vi "Job (Caraya Test).vi"() -> ()   [LabVIEW 2013]
uses:
  <vilib>/LabVIEW Open Source Project/Cron Scheduler/Job/Job.lvclass
  Caraya Job Configuration -- cluster.ctl
  <vilib>/LabVIEW Open Source Project/Cron Scheduler/Job/Job.lvclass/Job.ctl
  <vilib>/LabVIEW Open Source Project/Cron Scheduler/Job/Read Abort Notifier.vi
  <vilib>/addons/_JKI Toolkits/Caraya/run-tests/Run Test (Scalar Path).vi
  <vilib>/addons/_JKI Toolkits/Caraya/Caraya.lvlib
  <vilib>/addons/_JKI.lib/Serialization/JSON/JKI JSON Serialization.lvlib
panel:
  out "Test Configuration":T1={"Test Path"=path "", "Report Path"=path "", "Inspect Recursively"=TRUE, "Verbose"=TRUE}
  out "Job out":refnum<class "Job.lvclass">
  out "error out":errorcluster
  in  "Job":refnum<class "Job.lvclass">
  out "stdout":string
  in  "stdin":string
  # "Macro: Initialize\nList the tasks to be execute for this job\n\nThere are two ways to terminate the job: \n1- Call the \"Macro: Exit\" state at the end of your task execution.\n2- Comment out the \"Macro: Exit\" state in \"Macro: Initialize\" case and monitor a Job completion condition instead. Use the \"Action: Check Job Complete\" state to instruct the job to terminate.\n\nAction: Read Standard Input\nUse this case to read the stdin terminal and initialize your job.\n\nAction: Write Standard Output\nMake sure to write your return value to the stdout terminal before exiting this VI."
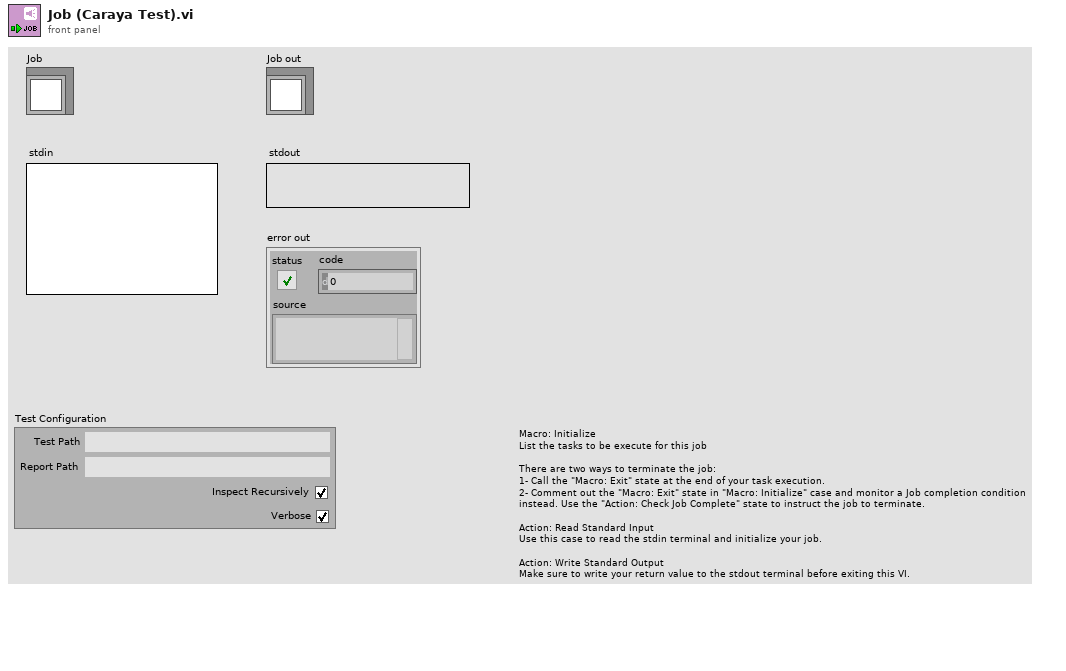
[diagram p1: front panel]
types:
  T1 = typedef "Caraya Job Configuration -- cluster.ctl" = cluster{"Test Path":path, "Report Path":path, "Inspect Recursively":bool, "Verbose":bool}
  T2 = enum32{"Invalid", "Standard", "Closed", "Hidden", "Minimized", "Maximized"}
  T3 = enum32{"invalid app kind", "Development System", "Run Time System", "Student Edition", "Embedded LabVIEW", "Evaluation", "Custom"}
  T4 = cluster{"Core":cluster{"Current VI Reference":refnum<vi>, "Close Panel on Exit?":bool}, "Job":refnum<class "Job.lvclass">, "stdin":string, "stdout":string, "stderror":errorcluster, "start time":timestamp, "Test Configuration":T1}
  T5 = cluster{"Current VI Reference":refnum<vi>, "Close Panel on Exit?":bool}
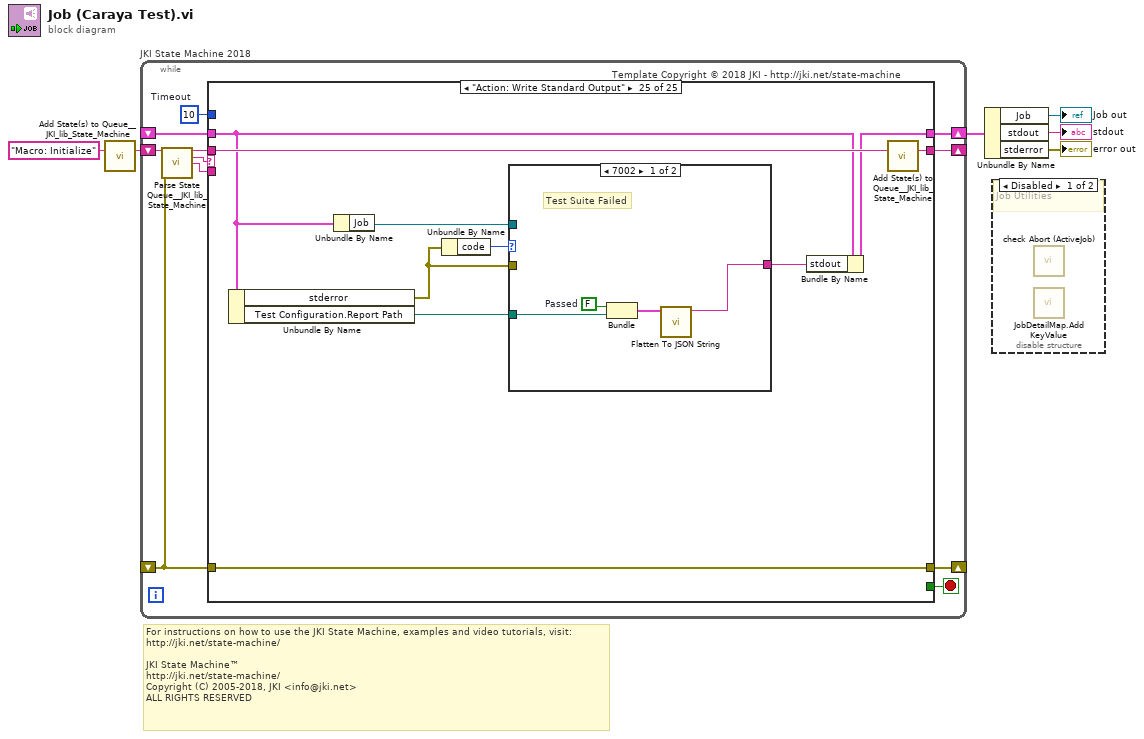
[diagram p0: block diagram]
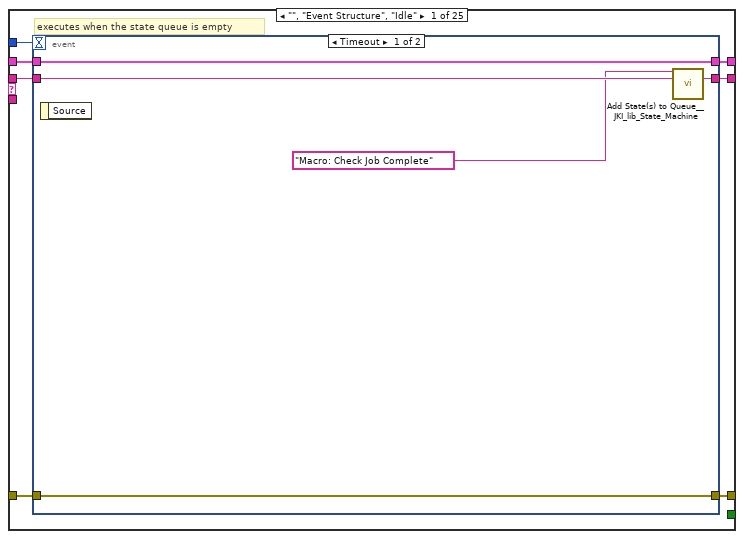
[diagram p3: hidden frame]
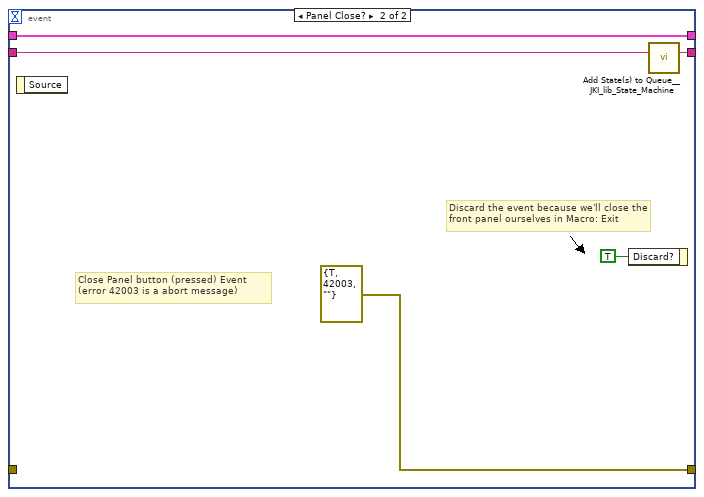
[diagram p4: hidden frame]
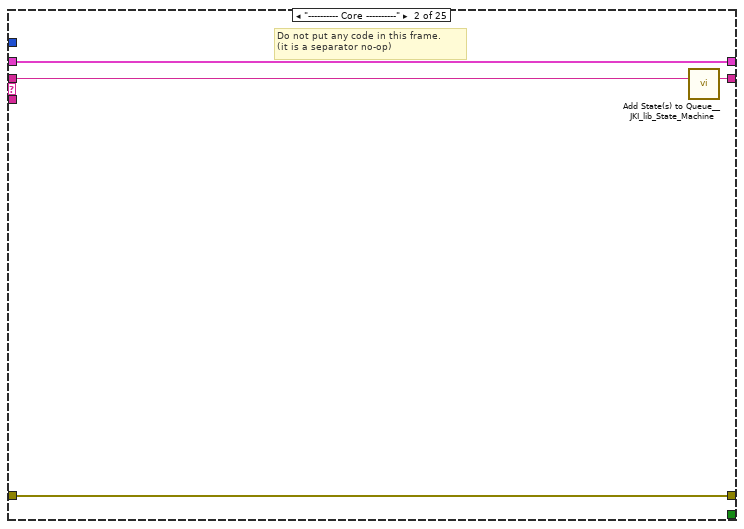
[diagram p5: hidden frame]
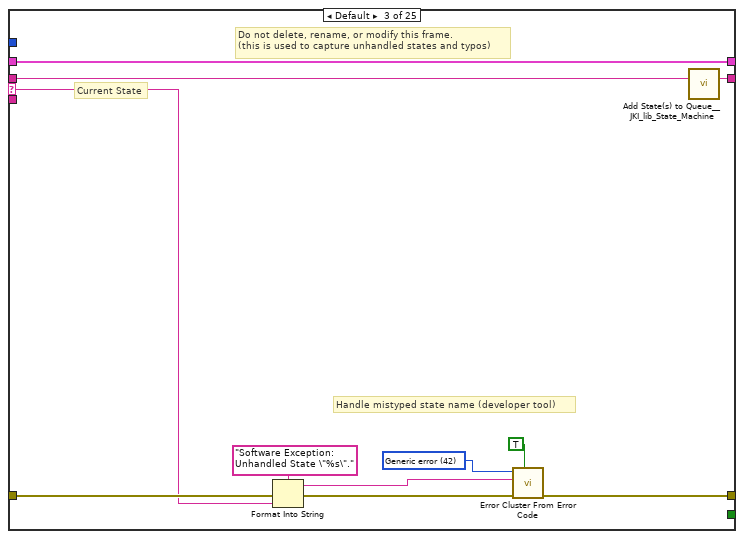
[diagram p6: hidden frame]
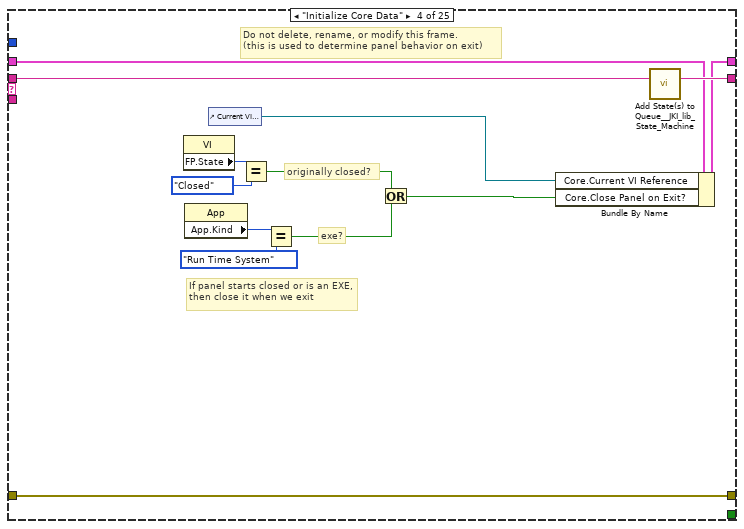
[diagram p7: hidden frame]
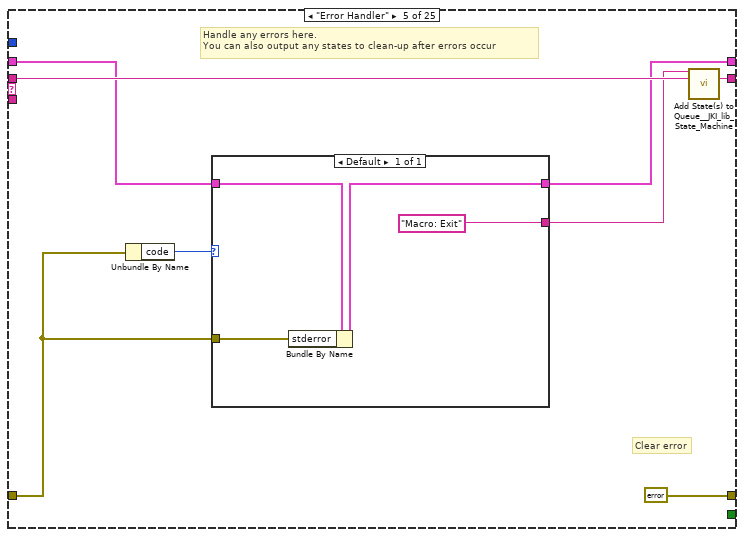
[diagram p8: hidden frame]
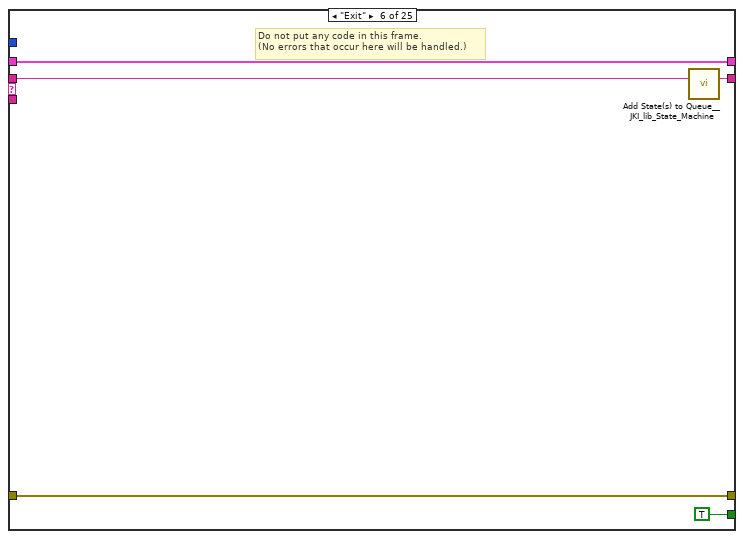
[diagram p9: hidden frame]
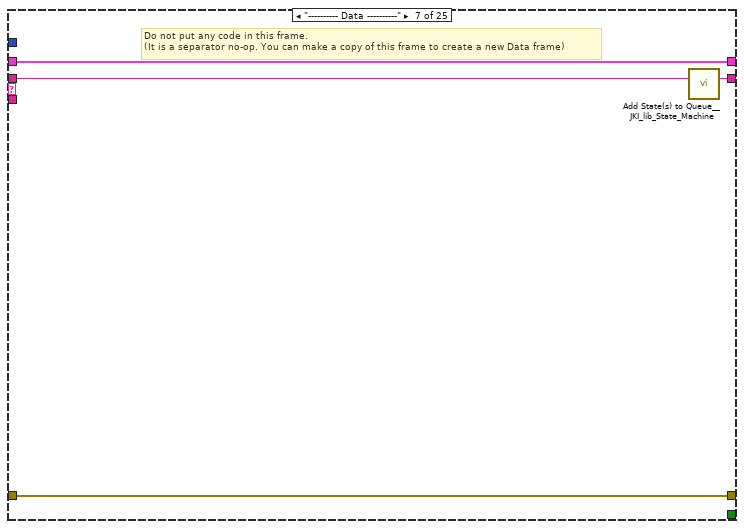
[diagram p10: hidden frame]
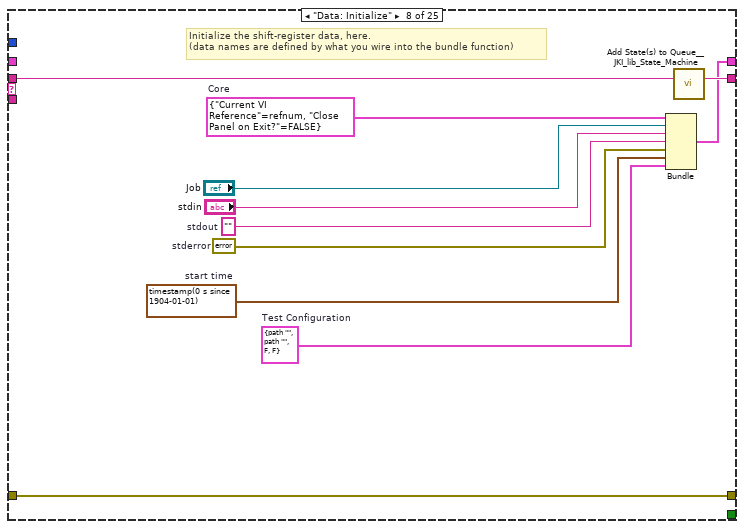
[diagram p11: hidden frame]
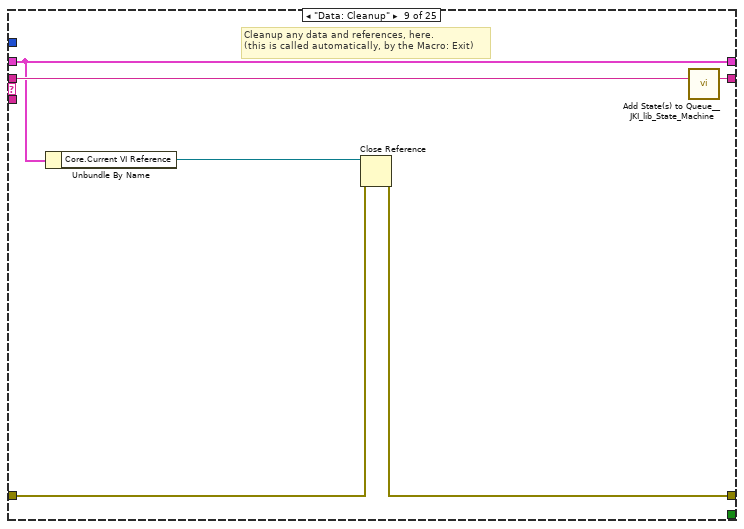
[diagram p12: hidden frame]
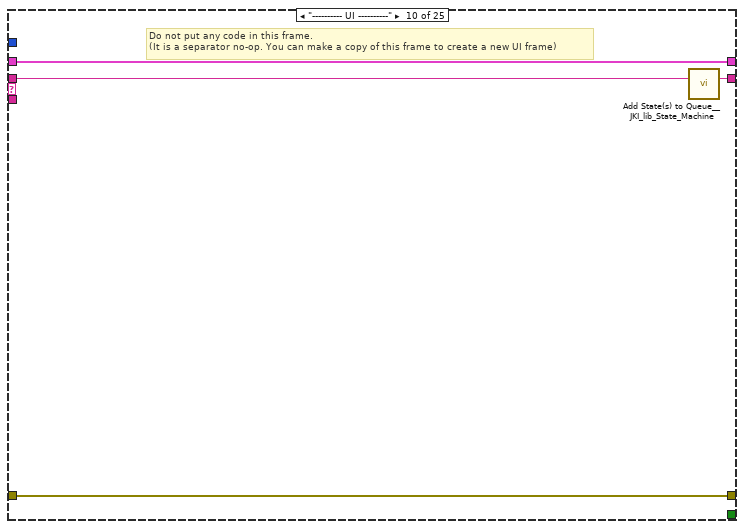
[diagram p13: hidden frame]
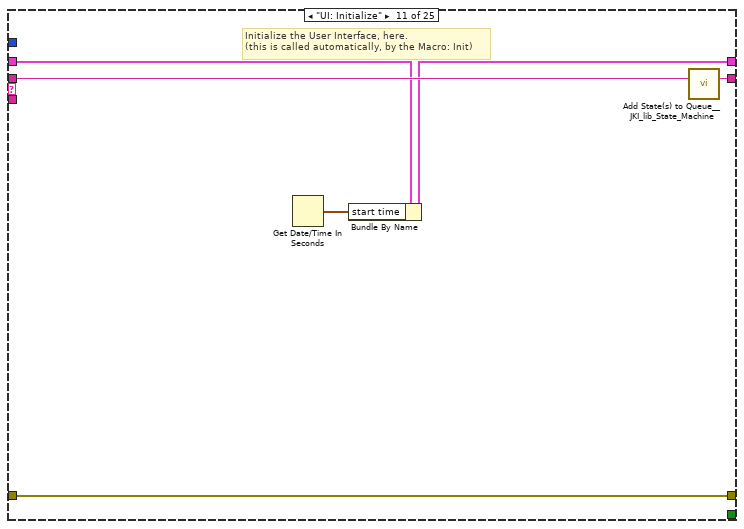
[diagram p14: hidden frame]
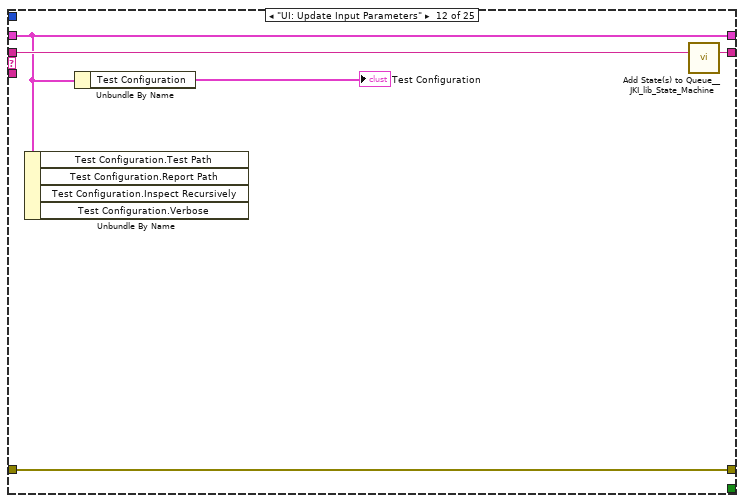
[diagram p15: hidden frame]
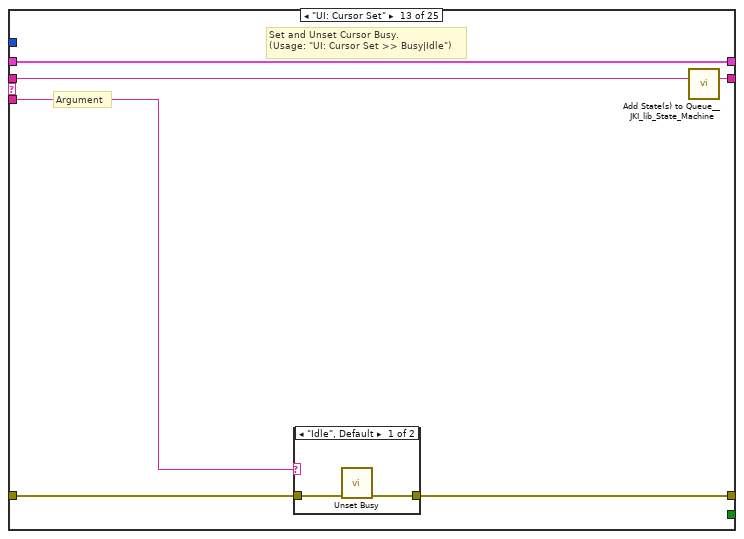
[diagram p16: hidden frame]
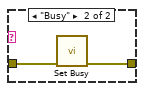
[diagram p17: hidden frame]
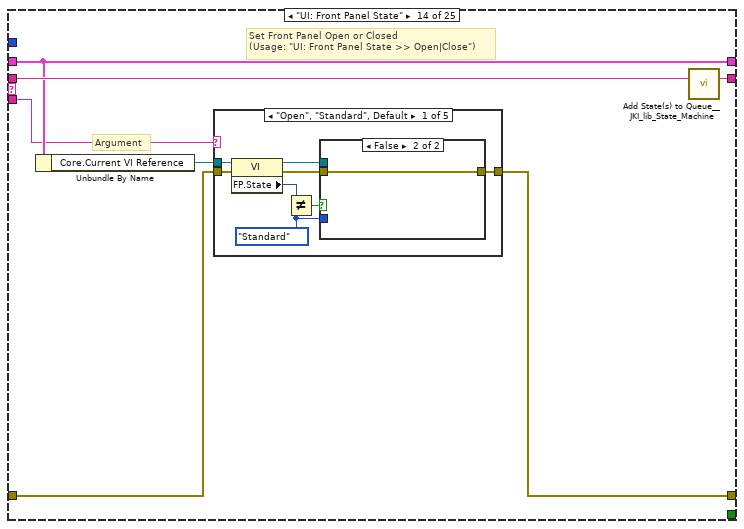
[diagram p18: hidden frame]
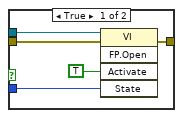
[diagram p19: hidden frame]
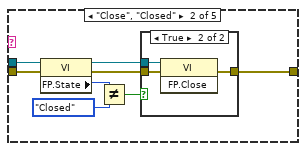
[diagram p20: hidden frame]
diagram:
  # "For instructions on how to use the JKI State Machine, examples and video tutorials, visit:\nhttp://jki.net/state-machine/\n\nJKI State Machine™\nhttp://jki.net/state-machine/\nCopyright (C) 2005-2018, JKI <info@jki.net>\nALL RIGHTS RESERVED"
  n1 = call <vilib>:"Add State(s) to Queue__JKI_lib_State_Machine.vi"("State(s) in (\"\")"="Macro: Initialize") -> ("States Out"=w6:string)  [unwired: 14 in]
  n2 = while "JKI State Machine 2018" {
    shift-right: [w10] -> w4
    shift-left: _ -> [w9]
    shift-right: [w13] -> _
    shift-left: _ -> [w7]
    shift-right: [w12] -> _
    shift-left: w6 -> [w14]
    stop <- w11 stop-if-true
    w8 = 10  # Timeout
    # "Template Copyright © 2018 JKI - http://jki.net/state-machine"
    n3 = call <vilib>:"Parse State Queue__JKI_lib_State_Machine.vi"("State Queue"=w14, "Error In (no error)"=w7) -> ("Remaining States"=w16:string, "Current State"=w17:string, "Arguments"=w15:string)  [unwired: 11 in]
    n4 = case shown="\"Action: Write Standard Output\"" w17 {
      selector: w17 -> [_ _ w39 _ _ _ _ _ _ _ _ _ _ _ _ _ _ _ _ w244 _ _ _ _ _]
      tunnel: w16 -> [w24 w38 w43 w62 w70 w79 w83 w94 w100 w104 w110 w115 w121 w132 w201 w206 w211 w222 w228 w248 w262 w272 w282 w307 w317]
      tunnel: w15 -> [_ _ _ _ _ _ _ _ _ _ _ _ w116 w126 _ _ _ _ _ _ _ _ _ _ _]
      tunnel: w9 -> [w22 w35 w41 w55 w65 w77 w80 _ w95 w101 w106 w112 w119 w128 w198 w203 w208 w219 w225 w242 w254 w270 w280 w305 w311]
      tunnel: [w21 w36 w45 w59 errorcluster {"status"=FALSE, "code"=0, "source"=""} ("error out") w76 w81 w91 w96 w102 w108 w113 w117 w129 w199 w204 w209 w220 w226 w229 w260 w264 w274 w288 w315] -> w13
      tunnel: w7 -> [w20 w36 w44 w59 w66 w76 w81 w91 w97 w102 w108 w113 w118 w130 w199 w204 w209 w220 w226 w233 w260 w263 w275 w283 w315]
      tunnel: [w23 w37 w42 w61 w69 w78 w82 w93 w99 w103 w109 w114 w120 w131 w200 w205 w210 w221 w227 w247 w261 w271 w281 w306 w316] -> w12
      tunnel: [_ _ _ _ _ TRUE _ _ _ _ _ _ _ _ _ _ _ _ _ _ _ _ _ _ _] -> w11
      tunnel: [w19 w35 w41 w60 w64 w77 w80 w92 w95 w101 w105 w112 w119 w128 w198 w203 w208 w219 w224 w246 w259 w269 w279 w304 w314] -> w10
      tunnel: w8 -> [w18 _ _ _ _ _ _ _ _ _ _ _ _ _ _ _ _ _ _ _ _ _ _ _ _]
      frame "", "Event Structure", "Idle" {
        # "executes when the state queue is empty"
        n5 = event shown="[0] Timeout" {
          selector: _ -> [_ _]
          dyn-events: _ -> [_ _]
          timeout: w18 -> [_ _]
          tunnel: w24 -> [w29 w34]
          tunnel: [w28 w33] -> w23
          tunnel: w22 -> [w26 w32]
          tunnel: [w27 errorcluster {"status"=TRUE, "code"=42003, "source"=""} ("error constant")] -> w21
          tunnel: w20 -> [w27 _]
          tunnel: [w26 w32] -> w19
          event Timeout {
            n6 = event-data() -> ()  [unwired: 1 in, 1 out]
            n7 = call <vilib>:"Add State(s) to Queue__JKI_lib_State_Machine.vi"("State(s) in Front (\"\")"="Macro: Check Job Complete", "State(s) in (\"\")"=w29) -> ("States Out"=w28:string)  [unwired: 13 in]
          }
          event Panel Close? {
            # "Discard the event because we'll close the front panel ourselves in Macro: Exit"
            # "Close Panel button (pressed) Event\n(error 42003 is a abort message)"
            n8 = event-data() -> ()  [unwired: 1 in, 1 out]
            n9 = event-data("Discard?"=TRUE) -> ()  [unwired: 1 in, 1 out]
            n10 = call <vilib>:"Add State(s) to Queue__JKI_lib_State_Machine.vi"("State(s) in (\"\")"=w34) -> ("States Out"=w33:string)  [unwired: 14 in]
          }
        }
      }
      frame "---------- Core ----------" {
        # "Do not put any code in this frame.\n(it is a separator no-op)"
        n11 = call <vilib>:"Add State(s) to Queue__JKI_lib_State_Machine.vi"("State(s) in (\"\")"=w38) -> ("States Out"=w37:string)  [unwired: 14 in]
      }
      frame Default {
        w48 = 42 items=["No error", "Argument error", "Memory is full", "Out of zone", "End of file", "File already open", "Generic file I/O error", "File not found", "File permission error", "Disk is full", "Duplicate path", "Too many files open", "System feature not enabled", "Resource file not found", "Cannot add resource", "Resource not found", "Image not found", "Image memory error", "Pen does not exist", "Config type invalid", "Config token not found", "Config parse error", "Config memory error", "Bad external code format", "Bad external code offset", "External code not present", "Null window", "Destroy window error", "Null menu", "Print aborted", "Bad print record", "Print driver error", "Windows error during printing", "Memory error during printing", "Print dialog error", "Generic print error", "Invalid device refnum", "Device not found", "Device parameter error", "Device unit error", "Cannot open device", "Device call aborted", "Generic error", "Cancelled by user", "Object ID too low", "Object ID too high", "Object not in heap", "Unknown heap", "Unknown object (invalid DefProc)", "Unknown object (DefProc not in table)", "Message out of range", "Invalid (null) method", "Unknown message", "Manager call not supported", "Bad address", "Network operation in progress", "Network operation timed out", "Connection is busy", "Network attribute not supported", "Network error", "Address in use", "System out of memory", "Connection aborted", "Connection refused", "Not connected", "Already connected", "Connection closed", "Initialization error (interapplication manager)", "Bad occurrence", "Wait on unbound occurrence handler", "Occurrence queue overflow", "Datalog type conflict", "Unused", "Unrecognized type (interapplication manager)", "Memory corrupt", "Failed to make temporary DLL", "Old CIN version", "Drag socket not found", "Failed to load drop-object", "Failed to register OLE object", "Failed to release OLE object", "Format specifier type mismatch", "Unknown format specifier", "Too few format specifiers", "Too many format specifiers", "Scan failed", "Newer CIN version", "Error converting to variant", "Runtime menu error", "Password tampered", "Variant attribute not found", "Incompatible variant data type", "Event data is not available", "Event Store is not present", "Occurrence is not found", "Event Queue is not created", "Event info is not available", "Refnum passed is NULL", "Error retrieving Class GUID", "Error retrieving CoClass GUID", "Error retrieving TypeLib GUID.", "Bad built application magic bytes.", "Specific driver is different from the specific driver associated with the Logical Name.", "There is no session opened to the class driver.", "Max Error", "MAX - Error with config objects", "MAX - Error loading configuration", "MAX - Group not supported"]
        # "Current State"
        # "Do not delete, rename, or modify this frame.\n(this is used to capture unhandled states and typos)"
        # "Handle mistyped state name (developer tool)"
        n12 = Format Into String(format string="Software Exception: Unhandled State \"%s\"." ("message"), error in=w44, w39) -> (resulting string=w47:string, error out=w46:errorcluster)  [unwired: 1 in]
        n13 = call <vilib>:"Error Cluster From Error Code.vi"("show call chain? (False)"=TRUE, "error in (no error)"=w46, "error message (\"\")"=w47, "error code (0)"=w48) -> ("error out"=w45:errorcluster)  [unwired: 5 in]
        n14 = call <vilib>:"Add State(s) to Queue__JKI_lib_State_Machine.vi"("State(s) in (\"\")"=w43) -> ("States Out"=w42:string)  [unwired: 14 in]
      }
      frame "Initialize Core Data" {
        # "Do not delete, rename, or modify this frame.\n(this is used to determine panel behavior on exit)"
        # "originally closed?"
        # "exe?"
        # "If panel starts closed or is an EXE, then close it when we exit"
        n15 = property class="VI"() -> ("FP.State"=w52:T2)  [unwired: 2 in, 2 out]
        n16 = property class="App"() -> ("App.Kind"=w58:T3)  [unwired: 2 in, 2 out]
        n17 = control-ref of="Current VI Reference"() -> (w53:refnum<vi>)
        n18 = Equal?(x=w52, y=T2."Closed" ("Front Panel Window:State")) -> (x = y?=w50:bool)
        n19 = Equal?(x=w58, y=T3."Run Time System" ("Application:Kind")) -> (x = y?=w56:bool)
        n20 = Or(x=w50, y=w56) -> (x .or. y?=w54:bool)
        n21 = Bundle By Name(cluster=w55, "Core.Current VI Reference"=w53, "Core.Close Panel on Exit?"=w54) -> (w60:T4)
        n22 = call <vilib>:"Add State(s) to Queue__JKI_lib_State_Machine.vi"("State(s) in (\"\")"=w62) -> ("States Out"=w61:string)  [unwired: 14 in]
      }
      frame "Error Handler" {
        # "Handle any errors here.\nYou can also output any states to clean-up after errors occur"
        # "Clear error"
        n23 = Unbundle By Name(w66) -> ("code"=w67:i32)
        n24 = case shown="Default" w67 {
          tunnel: w66 -> [w73]
          tunnel: w65 -> [w74]
          tunnel: [w72] -> w64
          tunnel: ["Macro: Exit"] -> w63
          frame Default {
            n25 = Bundle By Name(cluster=w74, "stderror"=w73) -> (w72:T4)
          }
        }
        n26 = call <vilib>:"Add State(s) to Queue__JKI_lib_State_Machine.vi"("State(s) in Front (\"\")"=w63, "State(s) in (\"\")"=w70) -> ("States Out"=w69:string)  [unwired: 13 in]
      }
      frame "Exit" {
        # "Do not put any code in this frame.\n(No errors that occur here will be handled.)"
        n27 = call <vilib>:"Add State(s) to Queue__JKI_lib_State_Machine.vi"("State(s) in (\"\")"=w79) -> ("States Out"=w78:string)  [unwired: 14 in]
      }
      frame "---------- Data ----------" {
        # "Do not put any code in this frame.\n(It is a separator no-op. You can make a copy of this frame to create a new Data frame)"
        n28 = call <vilib>:"Add State(s) to Queue__JKI_lib_State_Machine.vi"("State(s) in (\"\")"=w83) -> ("States Out"=w82:string)  [unwired: 14 in]
      }
      frame "Data: Initialize" {
        w84 = T1 {"Test Path"=path "", "Report Path"=path "", "Inspect Recursively"=FALSE, "Verbose"=FALSE}  # Test Configuration
        w85 = timestamp(0 s since 1904-01-01)  # start time
        w86 = errorcluster {"status"=FALSE, "code"=0, "source"=""}  # stderror
        w87 = ""  # stdout
        w90 = T5 {"Current VI Reference"=refnum, "Close Panel on Exit?"=FALSE}  # Core
        # "Initialize the shift-register data, here.\n(data names are defined by what you wire into the bundle function)"
        n29 = Bundle("Core"=w90, "Job"="Job", "stdin"="stdin", "stdout"=w87, "stderror"=w86, "start time"=w85, "Test Configuration"=w84) -> (w92:T4)  [unwired: 1 in]
        n30 = call <vilib>:"Add State(s) to Queue__JKI_lib_State_Machine.vi"("State(s) in (\"\")"=w94) -> ("States Out"=w93:string)  [unwired: 14 in]
      }
      frame "Data: Cleanup" {
        # "Cleanup any data and references, here.\n(this is called automatically, by the Macro: Exit)"
        n31 = Unbundle By Name(w95) -> ("Core.Current VI Reference"=w98:refnum<vi>)
        n32 = Close Reference(reference=w98, error in (no error)=w97) -> (error out=w96:errorcluster)
        n33 = call <vilib>:"Add State(s) to Queue__JKI_lib_State_Machine.vi"("State(s) in (\"\")"=w100) -> ("States Out"=w99:string)  [unwired: 14 in]
      }
      frame "---------- UI ----------" {
        # "Do not put any code in this frame.\n(It is a separator no-op. You can make a copy of this frame to create a new UI frame)"
        n34 = call <vilib>:"Add State(s) to Queue__JKI_lib_State_Machine.vi"("State(s) in (\"\")"=w104) -> ("States Out"=w103:string)  [unwired: 14 in]
      }
      frame "UI: Initialize" {
        # "Initialize the User Interface, here.\n(this is called automatically, by the Macro: Init)"
        n35 = Get Date/Time In Seconds() -> (seconds since 1Jan1904=w107:timestamp)
        n36 = Bundle By Name(cluster=w106, "start time"=w107) -> (w105:T4)
        n37 = call <vilib>:"Add State(s) to Queue__JKI_lib_State_Machine.vi"("State(s) in (\"\")"=w110) -> ("States Out"=w109:string)  [unwired: 14 in]
      }
      frame "UI: Update Input Parameters" {
        n38 = Unbundle By Name(w112) -> ()  [unwired: 4 out]
        n39 = Unbundle By Name(w112) -> ("Test Configuration"=→"Test Configuration":T1)
        n40 = call <vilib>:"Add State(s) to Queue__JKI_lib_State_Machine.vi"("State(s) in (\"\")"=w115) -> ("States Out"=w114:string)  [unwired: 14 in]
      }
      frame "UI: Cursor Set" {
        # "Argument"
        # "Set and Unset Cursor Busy.\n(Usage: \"UI: Cursor Set >> Busy|Idle\")"
        n41 = case shown="\"Idle\", Default" w116 {
          tunnel: w118 -> [w123 w125]
          tunnel: [w122 w124] -> w117
          frame "Idle", Default {
            n42 = call <vilib>:"Unset Busy.vi"("error in (no error)"=w123) -> ("error out"=w122:errorcluster)  [unwired: 10 in]
          }
          frame "Busy" {
            n43 = call <vilib>:"Set Busy.vi"("error in (no error)"=w125) -> ("error out"=w124:errorcluster)  [unwired: 9 in, 1 out]
          }
        }
        n44 = call <vilib>:"Add State(s) to Queue__JKI_lib_State_Machine.vi"("State(s) in (\"\")"=w121) -> ("States Out"=w120:string)  [unwired: 14 in]
      }
      frame "UI: Front Panel State" {
        # "Argument"
        # "Set Front Panel Open or Closed\n(Usage: \"UI: Front Panel State >> Open|Close\")"
        n45 = Unbundle By Name(w128) -> ("Core.Current VI Reference"=w127:refnum<vi>)
        n46 = case shown="\"Open\", \"Standard\", Default" w126 {
          tunnel: w130 -> [w138 w153 w164 w177 w190]
          tunnel: [w140 w154 w166 w179 w192] -> w129
          tunnel: w127 -> [w139 w151 w165 w178 w191]
          frame "Open", "Standard", Default {
            w133 = T2."Standard" ("State")
            n47 = property class="VI"(reference=w139, error in=w138) -> (reference out=w136:refnum<vi>, error out=w137:errorcluster, "FP.State"=w135:T2)
            n48 = Not Equal?(x=w135, y=w133) -> (x != y?=w134:bool)
            n49 = case shown="False" w134 {
              tunnel: [w144 w146] -> w140
              tunnel: w137 -> [w143 w146]
              tunnel: w136 -> [w142 _]
              tunnel: w133 -> [w141 _]
              frame True {
                n50 = invoke class="VI" method="FP.Open"(reference=w142, error in=w143, "Activate"=TRUE, "State"=w141) -> (error out=w144:errorcluster)  [unwired: 1 in, 4 out]
              }
              frame False {
              }
            }
          }
          frame "Close", "Closed" {
            n51 = property class="VI"(reference=w151, error in=w153) -> (reference out=w150:refnum<vi>, error out=w152:errorcluster, "FP.State"=w148:T2)
            n52 = Not Equal?(x=w148, y=T2."Closed" ("Front Panel Window:State")) -> (x != y?=w147:bool)
            n53 = case shown="True" w147 {
              tunnel: [w155 w158] -> w154
              tunnel: w152 -> [w155 w157]
              tunnel: w150 -> [_ w156]
              frame False {
              }
              frame True {
                n54 = invoke class="VI" method="FP.Close"(reference=w156, error in=w157) -> (error out=w158:errorcluster)  [unwired: 1 in, 2 out]
              }
            }
          }
          frame "Hidden", "Hide" {
            w159 = T2."Hidden" ("State")
            n55 = property class="VI"(reference=w165, error in=w164) -> (reference out=w162:refnum<vi>, error out=w163:errorcluster, "FP.State"=w161:T2)
            n56 = Not Equal?(x=w161, y=w159) -> (x != y?=w160:bool)
            n57 = case shown="True" w160 {
              tunnel: [w170 w171] -> w166
              tunnel: w163 -> [w169 w171]
              tunnel: w162 -> [w168 _]
              tunnel: w159 -> [w167 _]
              frame True {
                n58 = invoke class="VI" method="FP.Open"(reference=w168, error in=w169, "State"=w167) -> (error out=w170:errorcluster)  [unwired: 2 in, 4 out]
              }
              frame False {
              }
            }
          }
          frame "Minimize", "Minimized" {
            w172 = T2."Minimized" ("State")
            n59 = property class="VI"(reference=w178, error in=w177) -> (reference out=w175:refnum<vi>, error out=w176:errorcluster, "FP.State"=w174:T2)
            n60 = Not Equal?(x=w174, y=w172) -> (x != y?=w173:bool)
            n61 = case shown="True" w173 {
              tunnel: [w183 w184] -> w179
              tunnel: w176 -> [w182 w184]
              tunnel: w175 -> [w181 _]
              tunnel: w172 -> [w180 _]
              frame True {
                n62 = invoke class="VI" method="FP.Open"(reference=w181, error in=w182, "State"=w180) -> (error out=w183:errorcluster)  [unwired: 2 in, 4 out]
              }
              frame False {
              }
            }
          }
          frame "Maximize", "Maximized" {
            w185 = T2."Maximized" ("State")
            n63 = property class="VI"(reference=w191, error in=w190) -> (reference out=w188:refnum<vi>, error out=w189:errorcluster, "FP.State"=w187:T2)
            n64 = Not Equal?(x=w187, y=w185) -> (x != y?=w186:bool)
            n65 = case shown="True" w186 {
              tunnel: [w196 w197] -> w192
              tunnel: w189 -> [w195 w197]
              tunnel: w188 -> [w194 _]
              tunnel: w185 -> [w193 _]
              frame True {
                n66 = invoke class="VI" method="FP.Open"(reference=w194, error in=w195, "State"=w193) -> (error out=w196:errorcluster)  [unwired: 2 in, 4 out]
              }
              frame False {
              }
            }
          }
        }
        n67 = call <vilib>:"Add State(s) to Queue__JKI_lib_State_Machine.vi"("State(s) in (\"\")"=w132) -> ("States Out"=w131:string)  [unwired: 14 in]
      }
      frame "---------- Macro ----------" {
        # "Do not put any code in this frame.\n(It is a separator no-op. You can make a copy of this frame to create a new Macro frame)"
        n68 = call <vilib>:"Add State(s) to Queue__JKI_lib_State_Machine.vi"("State(s) in (\"\")"=w201) -> ("States Out"=w200:string)  [unwired: 14 in]
      }
      frame "Macro: Initialize" {
        w202 = "Data: Initialize\nInitialize Core Data\nUI: Initialize\nAction: Read Standard Input\nUI: Update Input Parameters\n\nUI: Front Panel State >> Open\n\n// Add your task actions below\nAction: Run Tests\n\nAction: Check Job Complete\n\n// Comment out the Macro: Exit line if you wish to exit on a condition\n// instead of exiting after a pre-determined action\n\n#Macro: Exit\n"  # Data: Initialize Initialize Core Data UI: Initialize Action: Read Standard Input UI: Update Input Parameters  UI: Front Panel State >> Open  // Add your task actions below Action: Run Tests  Action: Check Job Complete  // Comment out the Macro: Exit line if you wish to exit on a condition // instead of exiting after a pre-determined action  #Macro: Exit
        # "- Use the \"Action: Check Job Complete\" case to exit on a condition.\n- You can call Macro: Exit whenever you want to terminate the job.\n- Don't forget to set the Standard Output in the \"Action: Write Standard Output\" case if you wish to return results."
        # "Initialization Macro\n(This is called once, when the VI starts)"
        n69 = call <vilib>:"Add State(s) to Queue__JKI_lib_State_Machine.vi"("State(s) in Front (\"\")"=w202, "State(s) in (\"\")"=w206) -> ("States Out"=w205:string)  [unwired: 13 in]
      }
      frame "Macro: Check Job Complete" {
        # "Job Monitoring Macro\n(This is called regularly when the UI is idle)"
        n70 = call <vilib>:"Add State(s) to Queue__JKI_lib_State_Machine.vi"("State(s) in Front (\"\")"="Action: Check Job Complete\nAction: Check Abort", "State(s) in (\"\")"=w211) -> ("States Out"=w210:string)  [unwired: 13 in]
      }
      frame "Macro: Exit" {
        # "Exit Macro\n(This is called once, when the VI exits)"
        n71 = Unbundle By Name(w219) -> ("Core.Close Panel on Exit?"=w218:bool)
        n72 = Select(t="UI: Front Panel State >> Close", s=w218, f="") -> (s? t:f=w215:string)
        n73 = call <vilib>:"Add State(s) to Queue__JKI_lib_State_Machine.vi"("State(s) in Front (\"\")"="Action: Write Standard Output", "State(s) in (\"\")"=w215, "State(s) at Back (\"\")"="Data: Cleanup\nExit") -> ("States Out"=w213:string)  [unwired: 12 in]
        n74 = call <vilib>:"Add State(s) to Queue__JKI_lib_State_Machine.vi"("State(s) in Front (\"\")"=w213, "State(s) in (\"\")"=w222) -> ("States Out"=w221:string)  [unwired: 13 in]
      }
      frame "---------- Action ----------" {
        # "Action Separator\n(You can make a copy of, or modify, this frame)"
        n75 = Unbundle By Name(w225) -> ("Job"=w223:refnum<class "Job.lvclass">)  [unwired: 1 out]
        n76 = Bundle By Name(cluster=w225, "Job"=w223) -> (w224:T4)
        n77 = call <vilib>:"Add State(s) to Queue__JKI_lib_State_Machine.vi"("State(s) in (\"\")"=w228) -> ("States Out"=w227:string)  [unwired: 14 in]
      }
      frame "Action: Run Tests" {
        n78 = Unbundle By Name(w242) -> ("Job"=w245:refnum<class "Job.lvclass">)  [unwired: 1 out]
        n79 = Unbundle By Name(w242) -> ("Test Configuration.Report Path"=w237:path, "Test Configuration.Test Path"=w241:path, "Test Configuration.Inspect Recursively"=w239:bool, "Test Configuration.Verbose"=w238:bool)
        n80 = Get Date/Time In Seconds() -> (seconds since 1Jan1904=w243:timestamp)
        n81 = call <vilib>:"JobDetailMap.Add KeyValue.vi"("error in (no error)"=w233, "Value"=w243, "Key"=w244, "Job in"=w245) -> ("error out"=w232:errorcluster, "Job out"=w236:refnum<class "Job.lvclass">)  [unwired: 6 in]
        n82 = call-poly <vilib>:"Run Tests.vi"("Verbose"=w238, "Report Path"=w237, "Inspect Recursively (T)"=w239, "Test Path"=w241, "Interactive (T)"=FALSE) -> ("error out"=w230:errorcluster)  [unwired: 6 in]
        n83 = call <vilib>:"JobDetailMap.Add KeyValue.vi"("error in (no error)"=w232, "Value"=w230, "Key"="Post-Test Error", "Job in"=w236) -> ("error out"=w231:errorcluster, "Job out"=w235:refnum<class "Job.lvclass">)  [unwired: 6 in]
        n84 = Bundle By Name(cluster=w242, "Job"=w235) -> (w246:T4)
        n85 = Merge Errors(w231, w230) -> (w229:errorcluster)
        n86 = call <vilib>:"Add State(s) to Queue__JKI_lib_State_Machine.vi"("State(s) in (\"\")"=w248) -> ("States Out"=w247:string)  [unwired: 14 in]
      }
      frame "Action: Check Job Complete" {
        # "Terminates after a delay (demo).\nReplace with your own condition."
        n87 = Unbundle By Name(w254) -> ("Job"=w258:refnum<class "Job.lvclass">)
        n88 = Unbundle By Name(w254) -> ("start time"=w252:timestamp)
        n89 = Get Date/Time In Seconds() -> (seconds since 1Jan1904=w253:timestamp)
        n90 = Subtract(x=w253, y=w252) -> (x-y=w251:dbl)
        n91 = Bundle By Name(cluster=w254, "Job"=w258) -> (w259:T4)
        n92 = Greater Or Equal?(x=w251, y=3.0) -> (x >= y?=w249:bool)
        n93 = Select(t="Macro: Exit", s=w249, f="") -> (s? t:f=w255:string)
        n94 = call <vilib>:"Add State(s) to Queue__JKI_lib_State_Machine.vi"("State(s) in Front (\"\")"=w255, "State(s) in (\"\")"=w262) -> ("States Out"=w261:string)  [unwired: 13 in]
      }
      frame "Action: Check Abort" {
        n95 = Unbundle By Name(w270) -> ("Job"=w266:refnum<class "Job.lvclass">)  [unwired: 1 out]
        n96 = call <vilib>:"check Abort (ActiveJob).vi"("error in (no error)"=w263, "Job in"=w266) -> ("error out"=w267:errorcluster, "Abort"=w268:bool, "Job out"=w265:refnum<class "Job.lvclass">)  [unwired: 6 in, 1 out]
        n97 = Bundle By Name(cluster=w267, "status"=w268) -> (w264:errorcluster)
        n98 = Bundle By Name(cluster=w270, "Job"=w265) -> (w269:T4)
        n99 = call <vilib>:"Add State(s) to Queue__JKI_lib_State_Machine.vi"("State(s) in (\"\")"=w272) -> ("States Out"=w271:string)  [unwired: 14 in]
      }
      frame "Action: Update Map Data" {
        # "Use this pattern to add\nkey value pair data to the\nJob's map. This data is going\nto be available by the scheduler\nupon completion of the job."
        n100 = Unbundle By Name(w280) -> ("Job"=w278:refnum<class "Job.lvclass">)  [unwired: 1 out]
        n101 = Random Number (0-1)() -> (number: 0 to 1=w273:dbl)
        n102 = call <vilib>:"JobDetailMap.Add KeyValue.vi"("error in (no error)"=w275, "Value"=w273, "Key"="Value", "Job in"=w278) -> ("error out"=w274:errorcluster, "Job out"=w277:refnum<class "Job.lvclass">)  [unwired: 6 in]
        n103 = Bundle By Name(cluster=w280, "Job"=w277) -> (w279:T4)
        n104 = call <vilib>:"Add State(s) to Queue__JKI_lib_State_Machine.vi"("State(s) in (\"\")"=w282) -> ("States Out"=w281:string)  [unwired: 14 in]
      }
      frame "Action: Read Standard Input" {
        w292 = T1 {"Test Path"=path "", "Report Path"=path "", "Inspect Recursively"=FALSE, "Verbose"=FALSE}
        n105 = Unbundle By Name(w305) -> ("Job"=w303:refnum<class "Job.lvclass">, "stdin"=w296:string)
        n106 = call <vilib>:"Unflatten From JSON String.vi"("Nulls as Defaults (F)"=TRUE, "Type and Defaults"=w292, "error in (no error)"=w283, "JSON String"=w296) -> ("error out"=w294:errorcluster, "Variant"=w293:variant)  [unwired: 6 in]
        n107 = Variant To Data(error in=w294, type=w292, Variant=w293) -> (data=w291:T1, error out=w287:errorcluster)
        n108 = Unbundle By Name(w291) -> ("Test Path"=w300:path, "Report Path"=w299:path)
        n109 = Select(t="" ("Key"), s=w287, f="" ("Key")) -> (s? t:f=w284:string)
        n110 = call <vilib>:"JobDetailMap.Add KeyValue.vi"("Value"=w300, "Key"="Test Path", "Job in"=w303) -> ("error out"=w302:errorcluster, "Job out"=w301:refnum<class "Job.lvclass">)  [unwired: 7 in]
        n111 = call <vilib>:"JobDetailMap.Add KeyValue.vi"("error in (no error)"=w302, "Value"=w299, "Key"="Report Path", "Job in"=w301) -> ("error out"=w289:errorcluster, "Job out"=w297:refnum<class "Job.lvclass">)  [unwired: 6 in]
        n112 = Merge Errors(w283, w289) -> (w288:errorcluster)
        n113 = Bundle By Name(cluster=w305, "Job"=w297, "Test Configuration"=w291) -> (w304:T4)
        n114 = call <vilib>:"Add State(s) to Queue__JKI_lib_State_Machine.vi"("State(s) in Front (\"\")"=w284, "State(s) in (\"\")"=w307) -> ("States Out"=w306:string)  [unwired: 13 in]
      }
      frame "Action: Write Standard Output" {
        n115 = Unbundle By Name(w311) -> ("stderror"=w313:errorcluster, "Test Configuration.Report Path"=w308:path)
        n116 = Unbundle By Name(w311) -> ("Job"=w312:refnum<class "Job.lvclass">)
        n117 = Unbundle By Name(w313) -> ("code"=w309:i32)
        n118 = case shown="7002" w309 {
          selector: w309 -> [_ w329]
          tunnel: w313 -> [_ w332]
          tunnel: w312 -> [_ w331]
          tunnel: [w318 w330] -> w310
          tunnel: w308 -> [w319 w327]
          frame 7002 {
            w321 = FALSE  # Passed
            # "Test Suite Failed"
            n119 = Bundle("Passed"=w321, "Report Path"=w319) -> (w320:cluster{"Passed":bool, "Report Path":path})  [unwired: 1 in]
            n120 = call <vilib>:"Flatten To JSON String.vi"("Variant"=w320) -> ("JSON String"=w318:string)  [unwired: 9 in, 1 out]
          }
          frame Default {
            w328 = TRUE  # Passed
            n121 = call <vilib>:"Explain exception code.vi"("exception"=w329, "Job type"=w331) -> ("exception message"=w324:string)  [unwired: 7 in, 2 out]
            n122 = Bundle("Passed"=w328, "Report Path"=w327) -> (w326:cluster{"Passed":bool, "Report Path":path})  [unwired: 1 in]
            n123 = Bundle("exception message"=w324) -> (w323:cluster{"exception message":string})  [unwired: 1 in]
            n124 = call <vilib>:"Flatten To JSON String.vi"("Variant"=w323) -> ("JSON String"=w322:string)  [unwired: 9 in, 1 out]
            n125 = call <vilib>:"Flatten To JSON String.vi"("Variant"=w326) -> ("JSON String"=w325:string)  [unwired: 9 in, 1 out]
            n126 = Select(t=w322, s=w332, f=w325) -> (s? t:f=w330:string)
          }
        }
        n127 = Bundle By Name(cluster=w311, "stdout"=w310) -> (w314:T4)
        n128 = call <vilib>:"Add State(s) to Queue__JKI_lib_State_Machine.vi"("State(s) in (\"\")"=w317) -> ("States Out"=w316:string)  [unwired: 14 in]
      }
    }
  }
  n129 = Unbundle By Name(w4) -> ("Job"=→"Job out":refnum<class "Job.lvclass">, "stdout"=→"stdout":string, "stderror"=→"error out":errorcluster)
  n130 = disable-structure shown="Disabled" {
    frame Disabled {
      # "Job Utilities"
      n131 = call <vilib>:"check Abort (ActiveJob).vi"() -> ()  [unwired: 8 in, 4 out]
      n132 = call <vilib>:"JobDetailMap.Add KeyValue.vi"() -> ()  [unwired: 10 in, 2 out]
    }
    frame Enabled {
    }
  }
